vi "Default Instrument Setup.vi"(8 "error in (no error)":errorcluster, 11 "heater_parent in":refnum<class "heater_parent.lvclass">) -> (0 "error out":errorcluster, 3 "heater_parent out":refnum<class "heater_parent.lvclass">)   [LabVIEW 2020, in "polar_bear_plus_drivers.lvlib" / "heater_parent.lvclass"]
doc: "Sends a default command string to the instrument whenever a new VISA session is opened, or the instrument is reset. Use this VI as a subVI for the <b>Initialize</b> and <b>Reset</b> VIs. Altering this VI could cause these two VIs to operate incorrectly."
uses:
  <instrlib>/RxnRover/Driver Polar Bear Plus/heater_parent/heater_parent.lvclass
  <instrlib>/RxnRover/Driver Polar Bear Plus/heater_parent/heater_parent.lvclass/heater_parent.ctl
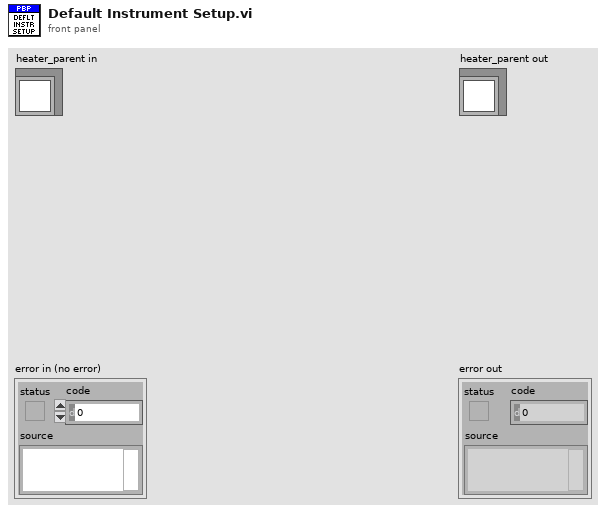
[diagram p1: front panel]
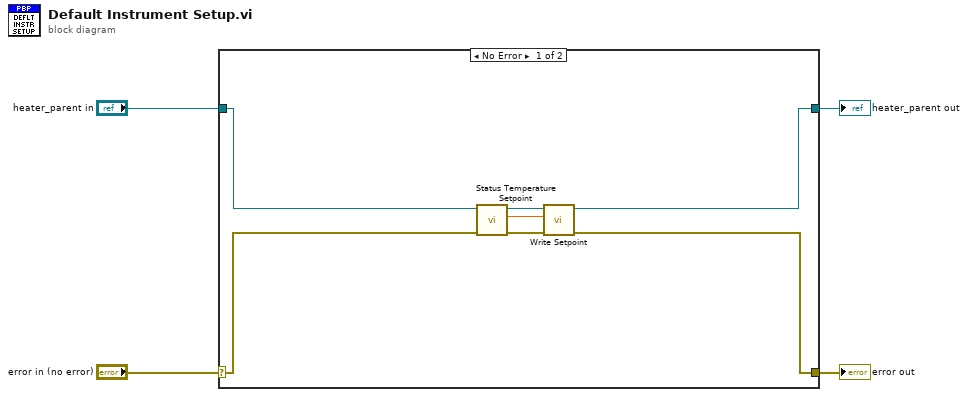
[diagram p0: block diagram]
diagram:
  n1 = case shown="No Error" "error in (no error)" {
    selector: "error in (no error)" -> [w11 w13]
    tunnel: [w8 w13] -> w3
    tunnel: [w6 w12] -> w1
    tunnel: "heater_parent in" -> [w9 w12]
    frame No Error {
      n2 = call-dynamic "Status Temperature Setpoint.vi"("error in (no error)"=w11, "heater_parent in"=w9) -> ("error out"=w10:errorcluster, "Setpoint"=w5:dbl, "heater_parent out"=w7:refnum<class "heater_parent.lvclass">)  [unwired: 7 in]
      n3 = call-dynamic "Write Setpoint.vi"("error in (no error)"=w10, "Setpoint"=w5, "heater_parent in"=w7) -> ("error out"=w8:errorcluster, "heater_parent out"=w6:refnum<class "heater_parent.lvclass">)  [unwired: 7 in]
    }
    frame Error {
    }
  }
  "error out" <- w3
  "heater_parent out" <- w1
